vi "getDevicePara.vi"(0 "Seetings in":T2, 1 "error in (no error)":errorcluster) -> (2 "Error Out":u32, 3 "Seetings out":T1, 4 "error out":errorcluster)   [LabVIEW 2021]
uses:
  <userlib>/er4commlib_labview/er4commlib_labview.lvlib
panel:
  out "prefix":u32
  out "realSamplingRate":dbl
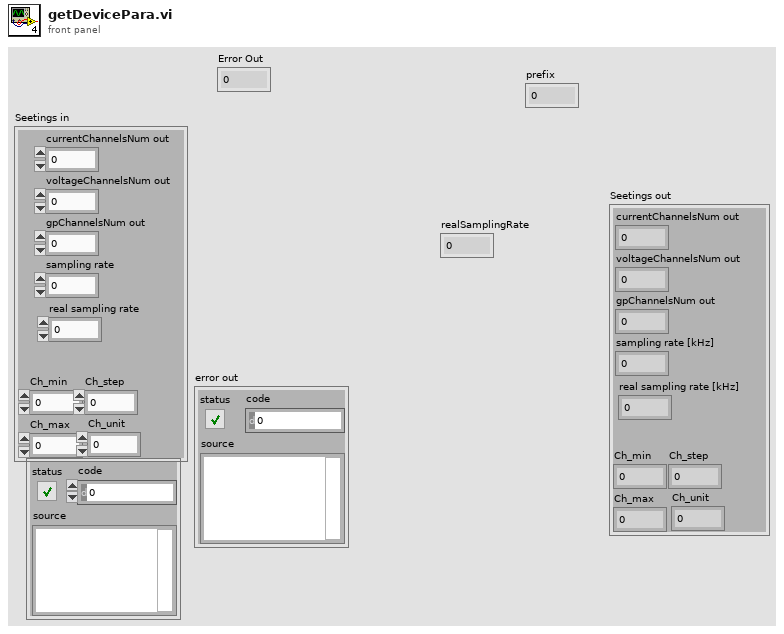
[diagram p1: front panel]
types:
  T1 = cluster{"currentChannelsNum out":u32, "voltageChannelsNum out":u32, "gpChannelsNum out":u32, "sampling rate [kHz]":dbl, "real sampling rate [kHz]":dbl, "Ch_min":dbl, "Ch_max":dbl, "Ch_step":dbl, "Ch_unit":dbl}
  T2 = cluster{"currentChannelsNum out":u32, "voltageChannelsNum out":u32, "gpChannelsNum out":u32, "sampling rate":dbl, "real sampling rate":dbl, "Ch_min":dbl, "Ch_max":dbl, "Ch_step":dbl, "Ch_unit":dbl}
  T3 = cluster{"min":dbl, "max":dbl, "step":dbl, "prefix":u32}
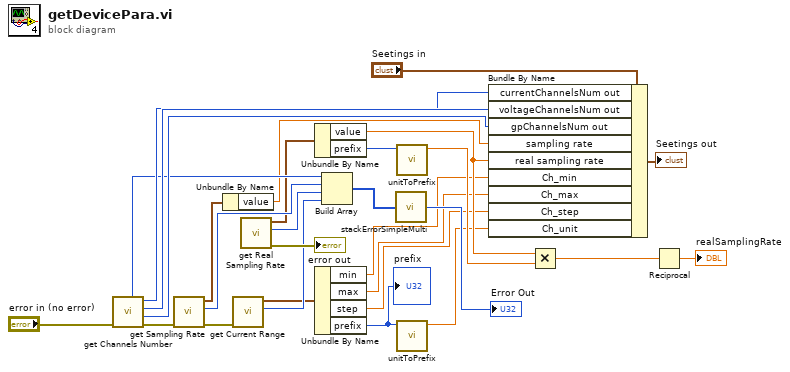
[diagram p0: block diagram]
diagram:
  n1 = call <userlib>:"get Channels Number.vi"("error in (no error)"="error in (no error)") -> ("error out"=w29:errorcluster, "gpChannelsNum out"=w23:u32, "currentChannelsNum out"=w22:u32, "voltageChannelsNum out"=w21:u32, "function return"=w18:u32)  [unwired: 6 in]
  n2 = call <userlib>:"get Sampling Rate.vi"("error in (no error)"=w29) -> ("error out"=w8:errorcluster, "function return"=w28:u32, "lvSamplingRate out"=w27:cluster{"value":dbl, "prefix":u32})  [unwired: 8 in]
  n3 = Unbundle By Name(w27) -> ("value"=w9:dbl)
  n4 = call <userlib>:"get Current Range.vi"("error in (no error)"=w8) -> ("function return"=w7:u32, "currentRange out"=w6:T3)  [unwired: 8 in, 1 out]
  n5 = call <userlib>:"get Real Sampling Rate.vi"() -> ("error out"=→"error out":errorcluster, "function return"=w13:u32, "samplingRate out"=w16:cluster{"value":dbl, "prefix":u32})  [unwired: 9 in]
  n6 = Unbundle By Name(w16) -> ("value"=w10:dbl, "prefix"=w15:u32)
  n7 = Unbundle By Name(w6) -> ("min"=w4:dbl, "max"=w3:dbl, "step"=w2:dbl, "prefix"=w5:u32)
  "prefix" <- w5
  n8 = Build Array(w18, w28, w13, w7) -> (w19:u32[])
  n9 = call "stackErrorSimpleMulti.vi"("Error List"=w19) -> ("Error Out"=→"Error Out":u32)
  n10 = call "unitToPrefix.vi"("prefix"=w15) -> ("Numeric"=w14:dbl)  [unwired: 10 in]
  n11 = call "unitToPrefix.vi"("prefix"=w5) -> ("Numeric"=w1:dbl)  [unwired: 10 in]
  n12 = Bundle By Name(cluster="Seetings in", "currentChannelsNum out"=w21, "voltageChannelsNum out"=w22, "gpChannelsNum out"=w23, "sampling rate"=w9, "real sampling rate"=w10, "Ch_min"=w4, "Ch_max"=w3, "Ch_step"=w2, "Ch_unit"=w1) -> (→"Seetings out":T2)
  n13 = Multiply(x=w10, y=w14) -> (x*y=w11:dbl)
  n14 = Reciprocal(x=w11) -> (1/x=→"realSamplingRate":dbl)
